vi "Query Output Lock State.vi"(8 "error in (no error)":errorcluster, 10 "Platform Slot Number (10)":i16=10 min=-1 max=255, 11 "VISA resource name":refnum<visa-resource-name>) -> (0 "error out":errorcluster, 2 "Shutter Lock State Enabled":bool, 3 "VISA resource name out":refnum<visa-resource-name>)   [LabVIEW 2018, in "LTB-1.lvlib" / "3150.lvlib"]
doc: "Queries the lock state of the instrument's shutter."
uses:
  3150.lvlib
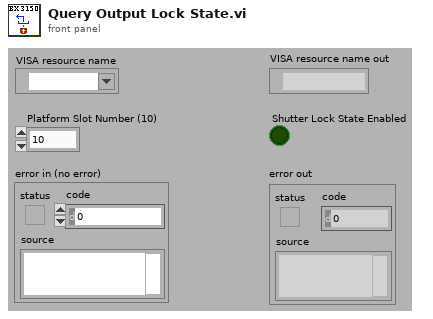
[diagram p1: front panel]
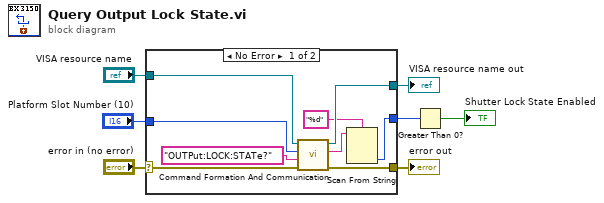
[diagram p0: block diagram]
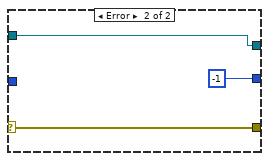
[diagram p2: hidden frame]
diagram:
  n1 = case shown="No Error" "error in (no error)" {
    selector: "error in (no error)" -> [w15 w18]
    tunnel: "VISA resource name" -> [w16 w19]
    tunnel: [w14 w19] -> w5
    tunnel: [w13 w18] -> w4
    tunnel: "Platform Slot Number (10)" -> [w11 _]
    tunnel: [w8 -1] -> w1
    frame No Error {
      n2 = call "Command Formation And Communication.vi"("error in (no error)"=w15, "Command"="OUTPut:LOCK:STATe?", "Platform Slot Number"=w11, "VISA resource name"=w16) -> ("error out"=w13:errorcluster, "Response"=w9:string, "VISA resource name out"=w14:refnum<visa-resource-name>)  [unwired: 1 in, 4 out]
      n3 = Scan From String(format string="%d", input string=w9) -> (output 1=w8:i32)  [unwired: 2 in, 4 out]
    }
    frame Error {
    }
  }
  "VISA resource name out" <- w5
  "error out" <- w4
  n4 = Greater Than 0?(x=w1) -> (x > 0?=→"Shutter Lock State Enabled":bool)
